vi "StrikerNormal.vi"(5 "Stop":bool, 6 "atacando ao contrário?":bool=TRUE, 7 "AI Parameters":T1={"GotoKick"={"Dist do cone a frente"=150.0, "attacker farback"=1500.0, "Perto"=300.0, "min dist to kick"=150.0, "kick eps"=0.0, "Time to transition"=0.05}, "Attacker"={"CC chute"=0.09, "CC passe"=0.045, "Kick Force"=100.0, "ball-robot Kick"=200.0, "ball-robot Pass"=0.3, "drible\nAttk"=FALSE}, "Defender"={"D max"=1700.0, "Vel p/ robô av"=1000.0, "Kick Force"=100.0, "D atk-def"=0.0, "D farback"=0.0, "drible\ndef"=FALSE, "drible\ngoalie"=FALSE}, "Timeout"={"Field/v in x"=6.0, "Dist Robots"=300, "Dist up in y"=300}, "Pose Striker"={"dist"=200.0, "Numeric"=-4.0, "dist 2"=200.0, "drible\nstriker"=FALSE}, "Dist Stop"=300.0, "D ball out"=200, "D central gap "=150.0, "T pass"=0.0, "Force ++"=0.0, "range kick"=0.0, "Chute alto"=TRUE, "Marcador novo"=TRUE, "drible"=FALSE, "D drible"=300.0} {"D drible" format="%#_13g"; "D central gap" format="%#_13g"; "Dist Stop" format="%#_13g"; "Pose Striker"."Numeric" format="%#_13g"; "Defender"."Kick Force" format="%#_13g"; "Defender"."Vel p/ robô av" format="%#_13g"; "Attacker"."ball-robot Kick" format="%#_13g"; "Attacker"."Kick Force" format="%#_13g"; "Attacker"."CC passe" format="%#_13g"; "Attacker"."CC chute" format="%#_13g"; "GotoKick"."kick eps" format="%#_13g"; "GotoKick"."min dist to kick" format="%#_13g"; "GotoKick"."Perto" format="%#_13g"; "GotoKick"."attacker farback" format="%#_13g"; "GotoKick"."Dist do cone a frente" format="%#_13g"}, 8 "IA Input":T9={"our_robots"=[], "enemy_robots"=[], "balls"=[], "geometry"={"line_width"=0, "field_length"=0, "field_width"=0, "boundary_width"=0, "referee_width"=0, "goal_width"=0, "goal_depth"=0, "goal_wall_width"=0, "center_circle_radius"=0, "defense_radius"=0, "defense_stretch"=0, "free_kick_from_defense_dist"=0, "penalty_spot_from_field_line_dist"=0, "penalty_line_from_spot_dist"=0}, "IA Judge"={"stage"="", "command"="", "our_goalie_id"=0.0, "enemy_goalie_id"=0.0, "command enum"=enum."Halt", "Time"=enum."Azul"}, "Received Timestamp"=timestamp(0 s since 1904-01-01), "Events"={"Touch"=FALSE, "Ball out"=FALSE, "id touch"=0.0, "Ball out of \nVision"=FALSE, "Ball inside \nGoalie area"=FALSE, "Robot not responding"=FALSE, "Robots responding status"=[1.0, 1.0, 1.0, 1.0, 1.0, 1.0], "Enemy Ball \nPossession"=FALSE, "Pass State"=FALSE, "id end of pass"=0.0, "Kick"=FALSE, "Id ini Possession"=0.0, "Ball Possesion"=FALSE, "Id Possesion"=0.0}}, 9 "balls":T7[](array[typedef])=[{"x"=-2165.869384765625, "y"=510.4085693359375, "timestamp"=timestamp(2082758857.4639893 s since 1904-01-01), "Vel_x"=0.0, "Vel_y"=0.0, "Pos Bola Est"=[]}], 10 "Field Size in":T8={"line_width"=10, "field_length"=6000, "field_width"=4000, "boundary_width"=250, "referee_width"=425, "goal_width"=700, "goal_depth"=180, "goal_wall_width"=20, "center_circle_radius"=500, "defense_radius"=500, "defense_stretch"=350, "free_kick_from_defense_dist"=700, "penalty_spot_from_field_line_dist"=450, "penalty_line_from_spot_dist"=350}, 11 "Robot in":T2={"id"=5, "function"=enum."Attacker", "x"=-1842.5054931640625, "y"=520.60986328125, "orientation"=-2.7555055618286133, "v_tangent"=0.0, "v_normal"=0.0, "v_ang"=0.0, "kick_x"=0.0, "kick_z"=0.0, "dribble"=FALSE, "Timestamp"=timestamp(2082758857.4639893 s since 1904-01-01), "estimatives"={"est_v_tangent"=0.0, "est_v_normal"=0.0, "est_vx"=0.0, "est_vy"=0.0, "Pos Robot Est"=[]}, "dest_x_kick"=0.0, "dest_y_kick"=0.0, "Gap Coord"=[], "States"=enum."GoToTangent", "Path "=[], "Path  Smooth"=[], "Dest"=[]}) -> (2 "Robot out":T2={"id"=5, "function"=enum."Attacker", "x"=-1842.5054931640625, "y"=520.60986328125, "orientation"=-2.7555055618286133, "v_tangent"=-0.08361641967936218, "v_normal"=-0.20513016702014014, "v_ang"=0.24456003022714357, "kick_x"=0.0, "kick_z"=0.0, "dribble"=FALSE, "Timestamp"=timestamp(2082758857.4639893 s since 1904-01-01), "estimatives"={"est_v_tangent"=0.0, "est_v_normal"=0.0, "est_vx"=0.0, "est_vy"=0.0, "Pos Robot Est"=[]}, "dest_x_kick"=0.0, "dest_y_kick"=0.0, "Gap Coord"=[], "States"=enum."GoToTangent", "Path "=[], "Path  Smooth"=[], "Dest"=[]})   [LabVIEW 2017]
uses:
  Core/AI Robot.ctl
  Functions Enum.ctl
  AttackerStates.ctl
  Path Planning/RRT/PathDests.ctl
  Path Planning/RRT/PathDest.ctl
  Core/AI Input.ctl
  Core/AI Ball.ctl
  Core/Field Size.ctl
  Core/AI Judge.ctl
  Command Enum.ctl
  Util/Events/Events.ctl
  AI Parameters.ctl
panel:
  in  "Wait pass perpendicular?":bool=TRUE
  in  "Marcador sempre":bool
  out "size(s)":i32
  in  "IDattacker":dbl
  in  "Yattacker":dbl
  in  "Xattacker":dbl
  out "States":T4
  out "sentido":dbl
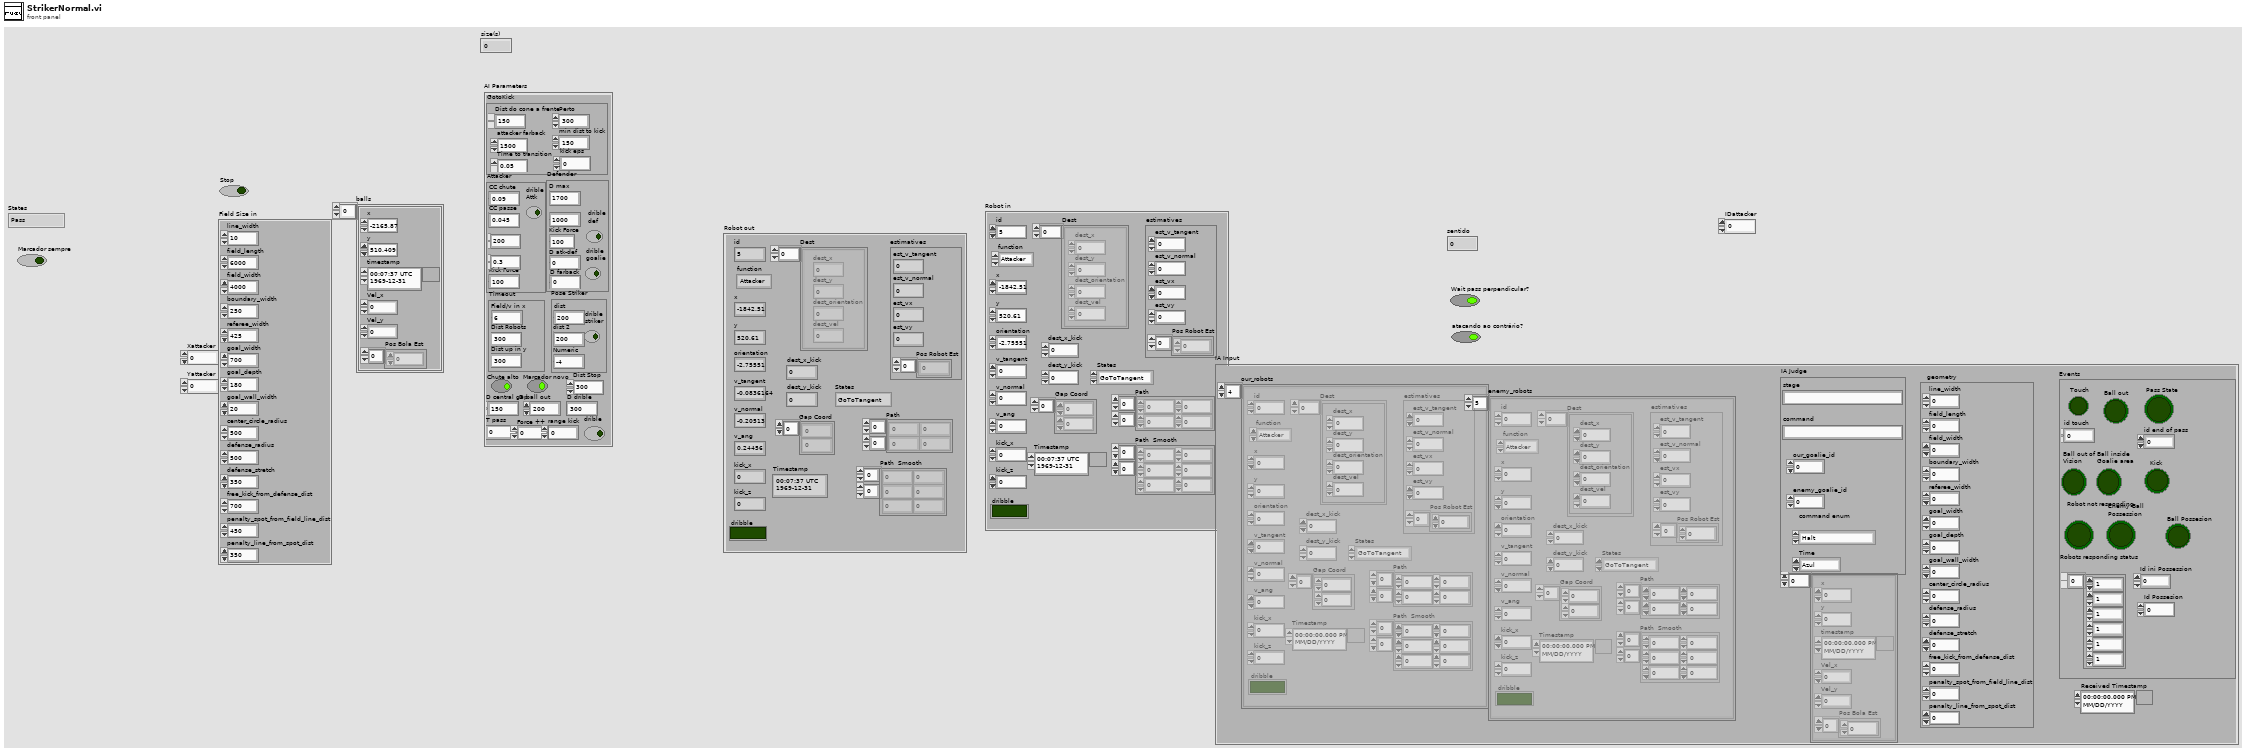
[diagram p1: front panel]
types:
  T1 = typedef "AI Parameters.ctl" = cluster{"GotoKick":cluster{"Dist do cone a frente":dbl, "attacker farback":dbl, "Perto":dbl, "min dist to kick":dbl, "kick eps":dbl, "Time to transition":dbl}, "Attacker":cluster{"CC chute":dbl, "CC passe":dbl, "Kick Force":dbl, "ball-robot Kick":dbl, "ball-robot Pass":dbl, "drible\nAttk":bool}, "Defender":cluster{"D max":dbl, "Vel p/ robô av":dbl, "Kick Force":dbl, "D atk-def":dbl, "D farback":dbl, "drible\ndef":bool, "drible\ngoalie":bool}, "Timeout":cluster{"Field/v in x":dbl, "Dist Robots":u32, "Dist up in y":u32}, "Pose Striker":cluster{"dist":dbl, "Numeric":dbl, "dist 2":dbl, "drible\nstriker":bool}, "Dist Stop":dbl, "D ball out":i32, "D central gap ":dbl, "T pass":dbl, "Force ++":dbl, "range kick":dbl, "Chute alto":bool, "Marcador novo":bool, "drible":bool, "D drible":dbl}
  T2 = typedef "AI Robot.ctl" = cluster{"id":u32, "function":T3, "x":dbl, "y":dbl, "orientation":dbl, "v_tangent":dbl, "v_normal":dbl, "v_ang":dbl, "kick_x":dbl, "kick_z":dbl, "dribble":bool, "Timestamp":timestamp, "estimatives":cluster{"est_v_tangent":dbl, "est_v_normal":dbl, "est_vx":dbl, "est_vy":dbl, "Pos Robot Est":dbl[]}, "dest_x_kick":dbl, "dest_y_kick":dbl, "Gap Coord":dbl[], "States":T4, "Path ":dbl[][], "Path  Smooth":dbl[][], "Dest":T5}
  T3 = typedef "Functions Enum.ctl" = enum16{"Attacker", "Goalie", "Defender", "Striker", "Goto 0", "Dummy", "Kicker", "ZigZag"}
  T4 = typedef "AttackerStates.ctl" = enum16{"Pass", "GoToTangent", "BallGetting", "GoToKick", ""}
  T5 = typedef "PathDests.ctl" = T6[]
  T6 = typedef "PathDest.ctl" = cluster{"dest_x":dbl, "dest_y":dbl, "dest_orientation":dbl, "dest_vel":dbl}
  T7 = typedef "AI Ball.ctl" = cluster{"x":dbl, "y":dbl, "timestamp":timestamp, "Vel_x":dbl, "Vel_y":dbl, "Pos Bola Est":dbl[]}
  T8 = typedef "Field Size.ctl" = cluster{"line_width":u32, "field_length":u32, "field_width":u32, "boundary_width":u32, "referee_width":u32, "goal_width":u32, "goal_depth":u32, "goal_wall_width":u32, "center_circle_radius":u32, "defense_radius":u32, "defense_stretch":u32, "free_kick_from_defense_dist":u32, "penalty_spot_from_field_line_dist":u32, "penalty_line_from_spot_dist":u32}
  T9 = typedef "AI Input.ctl" = cluster{"our_robots":T2[], "enemy_robots":T2[], "balls":T7[], "geometry":T8, "IA Judge":T10, "Received Timestamp":timestamp, "Events":T12}
  T10 = typedef "AI Judge.ctl" = cluster{"stage":string, "command":string, "our_goalie_id":dbl, "enemy_goalie_id":dbl, "command enum":T11, "Time":enum16{"Azul", "Amarelo"}}
  T11 = typedef "Command Enum.ctl" = enum16{"Halt", "Stop", "Force Start", "PKA Normal Start", "Prepare Kickoff Ally", "PKE Normal Start", "Prepare Kickoff Enemy", "Prepare Penalty Ally", "PPA Normal Start", "Prepare Penalty Enemy", "PPE Normal Start", "Direct Free Enemy", "Direct Free Ally", "Indirect Free Enemy", "Indirect Free Ally", "Timeout Enemy", "Timeout Ally", "Goal Enemy", "Goal Ally", "Ball Placement Enemy", "Ball Placement Ally", "Normal Half Time", "Extra Time Break", "Extra Half Time", "None", "Post Game"}
  T12 = typedef "Events.ctl" = cluster{"Touch":bool, "Ball out":bool, "id touch":dbl, "Ball out of \nVision":bool, "Ball inside \nGoalie area":bool, "Robot not responding":bool, "Robots responding status":dbl[], "Enemy Ball \nPossession":bool, "Pass State":bool, "id end of pass":dbl, "Kick":bool, "Id ini Possession":dbl, "Ball Possesion":bool, "Id Possesion":dbl}
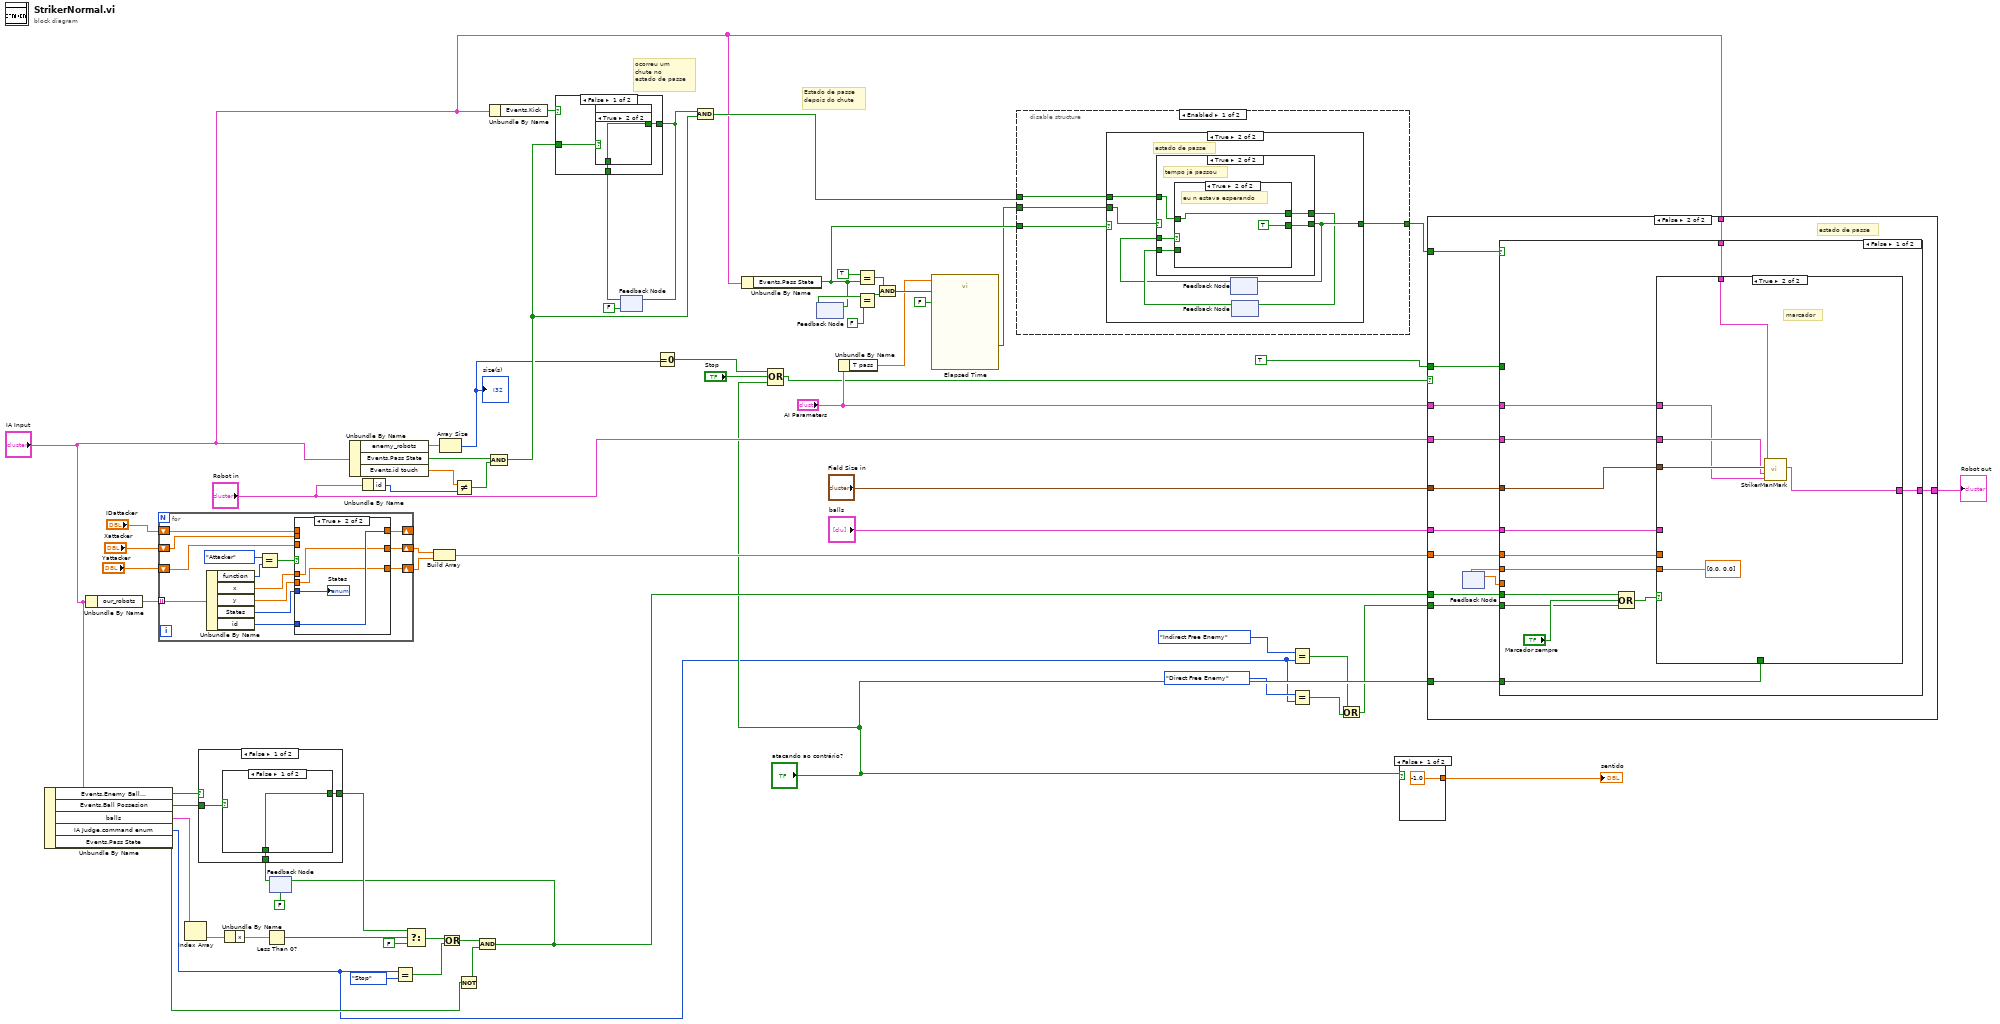
[diagram p0: block diagram]
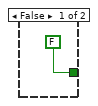
[diagram p2: hidden frame]
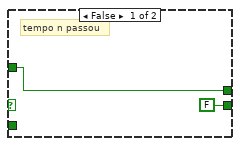
[diagram p3: hidden frame]
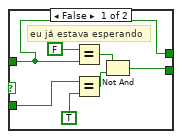
[diagram p4: hidden frame]
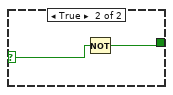
[diagram p6: hidden frame]
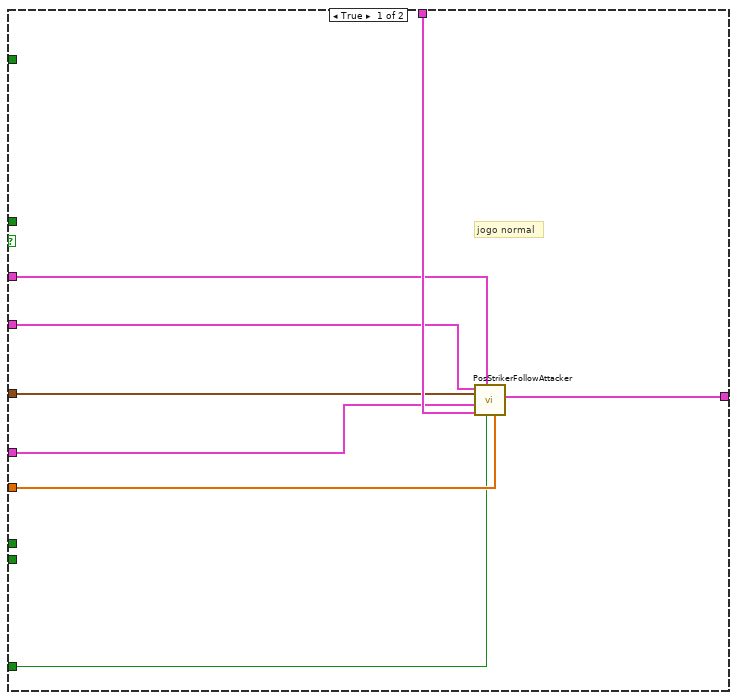
[diagram p8: hidden frame]
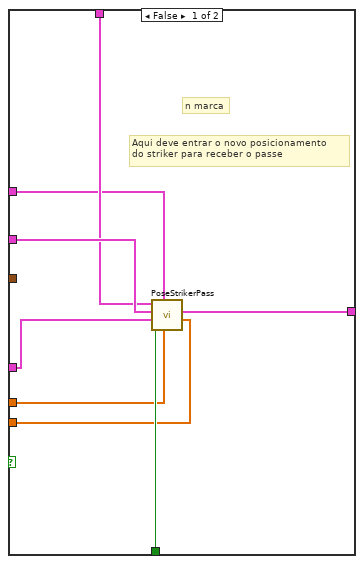
[diagram p9: hidden frame]
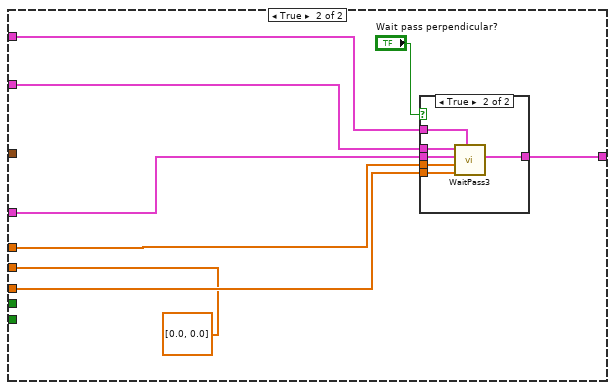
[diagram p10: hidden frame]
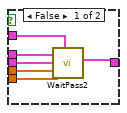
[diagram p11: hidden frame]
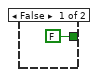
[diagram p13: hidden frame]
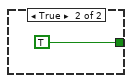
[diagram p14: hidden frame]
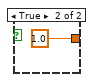
[diagram p15: hidden frame]
diagram:
  # "ocorreu um \nchute no\nestado de passe"
  # "Estado de passe\ndepois do chute"
  n1 = Unbundle By Name("IA Input") -> ("Events.Enemy Ball \nPossession"=w42:bool, "Events.Ball Possesion"=w41:bool, "balls"=w39:T7[], "IA Judge.command enum"=w4:T11, "Events.Pass State"=w29:bool)
  n2 = Unbundle By Name("IA Input") -> ("our_robots"=w59:T2[])
  n3 = for {
    tunnel: w59 -> [w74] mode=indexing
    shift-right: [w70] -> w55
    shift-left: "Xattacker" -> [w68]
    shift-right: [w69] -> w54
    shift-left: "Yattacker" -> [w67]
    shift-right: [w71] -> _
    shift-left: "IDattacker" -> [w66]
    n4 = Unbundle By Name(w74) -> ("function"=w79:T3, "x"=w76:dbl, "y"=w75:dbl, "States"=w73:T4, "id"=w72:u32)
    n5 = Equal?(x=Functions_Enum."Attacker", y=w79) -> (x = y?=w77:bool)
    n6 = case shown="True" w77 {
      tunnel: w76 -> [_ w84]
      tunnel: w75 -> [_ w83]
      tunnel: w73 -> [_ w86]
      tunnel: w72 -> [_ w85]
      tunnel: [w80 w85] -> w71
      tunnel: [w82 w84] -> w70
      tunnel: [w81 w83] -> w69
      tunnel: w68 -> [w82 _]
      tunnel: w67 -> [w81 _]
      tunnel: w66 -> [w80 _]
      frame False {
      }
      frame True {
        "States" <- w86
      }
    }
  }
  n7 = Index Array(array=w39) -> (element=w38:T7)  [unwired: 1 in]
  n8 = Unbundle By Name(w38) -> ("x"=w37:dbl)
  n9 = Less Than 0?(x=w37) -> (x < 0?=w36:bool)
  n10 = feedback #1(FALSE) -> (w40:bool)
  n11 = case shown="False" w42 {
    selector: w42 -> [_ w93]
    tunnel: [w88 w93] -> w35
    tunnel: w41 -> [w89 _]
    tunnel: w40 -> [w87 _]
    frame False {
      n12 = case shown="False" w89 {
        selector: w89 -> [_ w91]
        tunnel: [w90 w92] -> w88
        tunnel: w87 -> [w90 _]
        frame False {
        }
        frame True {
          n13 = Not(x=w91) -> (.not. x?=w92:bool)
        }
      }
    }
    frame True {
    }
  }
  n14 = Unbundle By Name("IA Input") -> ("enemy_robots"=w14:T2[], "Events.Pass State"=w60:bool, "Events.id touch"=w48:dbl)
  n15 = Unbundle By Name("Robot in") -> ("id"=w47:u32)
  n16 = Equal?(x=w4, y=Command_Enum."Stop") -> (x = y?=w32:bool)
  n17 = Select(t=w35, s=w36, f=FALSE) -> (s? t:f=w33:bool)
  n18 = Build Array(w55, w54) -> (w53:dbl[])
  n19 = Array Size(array=w14) -> (size(s)=w12:i32)
  "size(s)" <- w12
  n20 = Or(x=w33, y=w32) -> (x .or. y?=w30:bool)
  n21 = Not Equal?(x=w48, y=w47) -> (x != y?=w49:bool)
  n22 = Not(x=w29) -> (.not. x?=w28:bool)
  n23 = And(x=w30, y=w28) -> (x .and. y?=w27:bool)
  n24 = feedback-in #1(w27) -> ()
  n25 = Unbundle By Name("IA Input") -> ("Events.Kick"=w64:bool)
  n26 = Compound Arithmetic op=AND(w60, w49) -> (w50:bool)
  n27 = feedback #2(FALSE) -> (w62:bool)
  n28 = case shown="False" w64 {
    tunnel: [w95 TRUE] -> w63
    tunnel: w62 -> [w94 _]
    tunnel: w50 -> [w96 _]
    frame False {
      n29 = case shown="True" w96 {
        tunnel: [FALSE w98] -> w95
        tunnel: w94 -> [_ w98]
        frame False {
        }
        frame True {
        }
      }
    }
    frame True {
    }
  }
  n30 = feedback-in #2(w63) -> ()
  n31 = Equal To 0?(x=w12) -> (x = 0?=w13:bool)
  n32 = And(x=w63, y=w50) -> (x .and. y?=w18:bool)
  n33 = Unbundle By Name("IA Input") -> ("Events.Pass State"=w16:bool)
  n34 = Compound Arithmetic op=OR(w13, "Stop", "atacando ao contrário?") -> (w9:bool)
  n35 = feedback #3() -> (w26:bool)  [unwired: 1 in]
  n36 = feedback-in #3(w16) -> ()
  n37 = Unbundle By Name("AI Parameters") -> ("T pass"=w10:dbl)
  n38 = Equal?(x=TRUE, y=w16) -> (x = y?=w22:bool)
  n39 = Equal?(x=w26, y=FALSE) -> (x = y?=w23:bool)
  n40 = And(x=w22, y=w23) -> (x .and. y?=w21:bool)
  n41 = call "Elapsed Time"("Time Target (s)"=w10, "Reset"=w21, "Auto Reset"=FALSE) -> ("Time has Elapsed"=w15:bool)  [unwired: 9 in, 7 out]
  n42 = disable-structure shown="Enabled" {
    disable-tunnel: w15 -> [w101 _]
    disable-tunnel: [w103 w127] -> w19
    disable-tunnel: w18 -> [w102 w127]
    disable-tunnel: w16 -> [w100 _]
    frame Enabled {
      n43 = case shown="True" w100 {
        tunnel: [FALSE w110] -> w103
        tunnel: w102 -> [_ w109]
        tunnel: w101 -> [_ w106]
        frame False {
        }
        frame True {
          # "estado de passe"
          n44 = feedback #4() -> (w105:bool)  [unwired: 1 in]
          n45 = feedback #5() -> (w107:bool)  [unwired: 1 in]
          n46 = case shown="True" w106 {
            tunnel: [FALSE w116] -> w110
            tunnel: w109 -> [w111 w115]
            tunnel: [w111 w113] -> w108
            tunnel: w107 -> [_ w114]
            tunnel: w105 -> [_ w117]
            frame False {
              # "tempo n passou"
            }
            frame True {
              # "tempo já passou"
              n47 = case shown="True" w117 {
                tunnel: [w119 TRUE] -> w116
                tunnel: w115 -> [w118 w125]
                tunnel: w114 -> [w120 _]
                tunnel: [w118 w125] -> w113
                frame False {
                  # "eu já estava esperando"
                  n48 = Equal?(x=FALSE, y=w118) -> (x = y?=w121:bool)
                  n49 = Equal?(x=w120, y=TRUE) -> (x = y?=w122:bool)
                  n50 = Not And(1:w122, 2:w121) -> (0:w119:bool)
                }
                frame True {
                  # "eu n estava esperando"
                }
              }
            }
          }
          n51 = feedback-in #4(w110) -> ()
          n52 = feedback-in #5(w108) -> ()
        }
      }
    }
    frame Disabled {
    }
  }
  n53 = Equal?(x=Command_Enum."Direct Free Enemy", y=w4) -> (x = y?=w3:bool)
  n54 = Equal?(x=Command_Enum."Indirect Free Enemy", y=w4) -> (x = y?=w2:bool)
  n55 = Compound Arithmetic op=OR(w2, w3) -> (w1:bool)
  n56 = case shown="False" "atacando ao contrário?" {
    tunnel: [-1.0 1.0] -> w65
    frame False {
    }
    frame True {
    }
  }
  "sentido" <- w65
  n57 = case shown="False" w9 {
    tunnel: w19 -> [_ w143]
    tunnel: TRUE -> [_ w144]
    tunnel: "Robot in" -> [w136 w151]
    tunnel: w53 -> [w133 w150]
    tunnel: "atacando ao contrário?" -> [w132 w149]
    tunnel: "Field Size in" -> [w135 w148]
    tunnel: "balls" -> [w134 w147]
    tunnel: "IA Input" -> [w137 w146]
    tunnel: [w131 w145] -> w51
    tunnel: "AI Parameters" -> [w130 w142]
    tunnel: w27 -> [_ w141]
    tunnel: w1 -> [_ w138]
    frame True {
      # "jogo normal"
      n58 = call "PosStrikerFollowAttacker.vi"("Pos Attacker"=w133, "atacando ao contrário?"=w132, "AI Parameters"=w130, "IA Input"=w137, "balls"=w134, "Field Size in"=w135, "Robot in"=w136) -> ("Robot out"=w131:T2)  [unwired: 4 in]
    }
    frame False {
      # "estado de passe"
      n59 = feedback #6() -> (w139:dbl[])  [unwired: 1 in]
      n60 = case shown="False" w143 {
        tunnel: w144 -> [_ _]
        tunnel: w151 -> [w163 w186]
        tunnel: w150 -> [w158 w185]
        tunnel: [w160 w184] -> w145
        tunnel: w149 -> [w164 _]
        tunnel: w148 -> [w157 _]
        tunnel: w147 -> [w162 w183]
        tunnel: w146 -> [w161 _]
        tunnel: w142 -> [w159 w179]
        tunnel: w141 -> [w156 _]
        tunnel: [w153 dbl[] [0.0, 0.0] ("FinalPosition")] -> w140
        tunnel: w139 -> [_ w182]
        tunnel: w138 -> [w152 _]
        frame False {
          n61 = Compound Arithmetic op=OR(w156, "Marcador sempre", w152) -> (w155:bool)
          n62 = case shown="True" w155 {
            tunnel: w164 -> [w172 _]
            tunnel: w163 -> [w171 w177]
            tunnel: w162 -> [w170 _]
            tunnel: w161 -> [w169 w175]
            tunnel: [w168 w176] -> w160
            tunnel: w159 -> [w167 w174]
            tunnel: w158 -> [w166 _]
            tunnel: w157 -> [_ w178]
            tunnel: [w165 dbl[] [0.0, 0.0] ("FinalPosition")] -> w153
            frame False {
              # "n marca"
              # "Aqui deve entrar o novo posicionamento\ndo striker para receber o passe"
              n63 = call "PoseStrikerPass.vi"("Array"=w166, "AI Parameters"=w167, "atacando ao contrário?"=w172, "balls"=w170, "Robot in"=w171, "IA Input"=w169) -> ("FinalPosition"=w165:dbl[], "Robot out"=w168:T2)  [unwired: 4 in]
            }
            frame True {
              # "marcador"
              n64 = call "StrikerManMark.vi"("AI Parameters"=w174, "Robot in"=w177, "Field Size in"=w178, "IA Input"=w175) -> ("Robot out"=w176:T2)  [unwired: 6 in, 1 out]
            }
          }
        }
        frame True {
          n65 = case shown="True" "Wait pass perpendicular?" {
            tunnel: w186 -> [w191 w198]
            tunnel: w185 -> [w189 w197]
            tunnel: [w192 w196] -> w184
            tunnel: w183 -> [w190 w195]
            tunnel: w182 -> [w188 w194]
            tunnel: w179 -> [w187 w193]
            frame False {
              n66 = call "WaitPass2.vi"("AI Parameters"=w187, "Best Y Inverso"=w188, "Target"=w189, "balls"=w190, "Robot in"=w191) -> ("Robot out"=w192:T2)  [unwired: 6 in]
            }
            frame True {
              n67 = call "WaitPass3.vi"("AI Parameters"=w193, "Best Y Inverso"=w194, "Target"=w197, "balls"=w195, "Robot in"=w198) -> ("Robot out"=w196:T2)  [unwired: 6 in]
            }
          }
        }
      }
      n68 = feedback-in #6(w140) -> ()
    }
  }
  "Robot out" <- w51
